vi "Create Channel.vi"(0 "Error Out":errorcluster, 5 "Maximum":dbl=5.0 format="%0.2f", 7 "Minimum":dbl=-5.0 format="%0.2f", 8 "Error In":errorcluster, 11 "Physical Channel":tag) -> (3 "Task Out":refnum<k21>)   [LabVIEW 2014]
uses:
  <vilib>/DAQmx/create/channels.llb/DAQmx Create Channel (AI-Voltage-Basic).vi
panel:
  # "Create Channel"
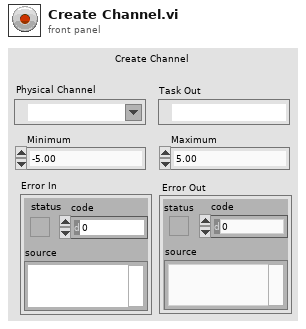
[diagram p1: front panel]
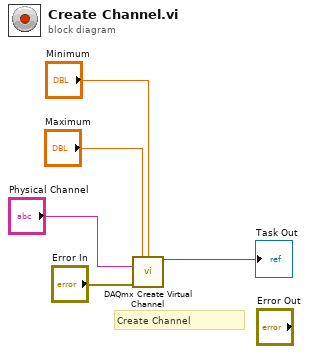
[diagram p0: block diagram]
diagram:
  # "Create Channel"
  n1 = call-poly <vilib>:"DAQmx Create Virtual Channel.vi"("maximum value"="Maximum", "minimum value"="Minimum", "physical channels"="Physical Channel", "error in"="Error In") -> ("task out"=→"Task Out":refnum<k21>)  [unwired: 10 in, 1 out]
